vi "Joystick 2 Disc Eject System.vi"(11 "Secondary Joystick Buttons":bool[](array[boolean])) -> (3 "Eject Disc":bool)   [LabVIEW 2018]
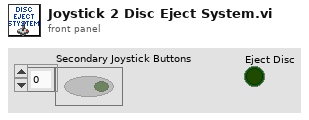
[diagram p1: front panel]
types:
  T1 = typedef "SecondaryJoystickButtons.ctl" = cluster{"Intake":bool, "Outtake":bool, "ShoulderMotor":bool, "ElbowMotor":bool, "Open Grip":bool, "Close Grip":bool, "Reset Arm Encoders":bool, "Eject Disc":bool}
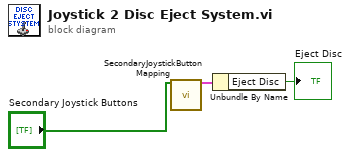
[diagram p0: block diagram]
diagram:
  n1 = call "SecondaryJoystickButtonMapping.vi"("Secondary joystick buttons"="Secondary Joystick Buttons") -> ("SecondaryJoystickButtons"=w3:T1)  [unwired: 13 in, 1 out]
  n2 = Unbundle By Name(w3) -> ("Eject Disc"=→"Eject Disc":bool)
